vi "Global 2.vi"() -> ()   [LabVIEW 2009]
panel:
  out "Present wavelength":dbl
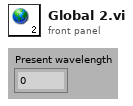
[diagram p1: front panel]
diagram:
